vi "Phase Tune.vi"(11 "Hardware Parameters":T1={"Scan Calibration [G/V]"=0.0, "Modulation Calibration [G/V]"=0.0, "Modulation Phase [deg]"=0.0, "Modulation Frequency [Hz]"=0.0, "Attenuation [dB]"=0, "Input Channel Count"=0, "Time constant"=7, "Sensitivity"=17, "Frequency Output Voltage [V]"=0.0, "Phase Output Voltage [V]"=0.0, "Lock-in Offset Compensation"=FALSE, "RF [GHz]"=0.0, "Q Start"=0.0, "Q End"=0.0, "Balance"=0.0, "Phase Error"=0.0, "AFC Error"=0.0, "AFC"=FALSE, "Magnet Rotation"=FALSE, "Balance Scaling Factor"=1.0, "Phase Error Scaling Factor"=1.0, "AFC Error Scaling Factor"=1.0, "Frequency Counter ID"="", "Sweep Waveform"=enum."Sawtooth", "Q-Factor Scale"=0.0, " Q-Data Scale"=0.0, " Q-Data Offset"=0.0, "Magnet Rotation Slope"=0.0, "Magnet Rotation Offset"=0.0, "Phase Sweep Resolution"=0.0, "Hardware Version Number"="", "Spectrometer ID Number"=0, "Spectrometer Name"="", "Lock in Saturation"=0.0, "Balance Threshold"=0.0, "Phase Error Threshold"=0.0, "AFC Error Threshold"=0.0, "Linear Actuator Length"=0.0, "Lock-in OK?"=FALSE, "Ignore Lock-in Comm. Failure"=FALSE, "Gradient Addresses"=[], "Gradient Calibrations [G/A*mm]"=[], "Gradient Power Supplies"=[], "Lock-in Address"="", "Magnet Type"=enum."RRI", "Camera Names"=[], "Sweep Limit [Gauss]"=0.0, "Modulation Limit [Gauss]"=0.0, "Balance Threshold Exceeded?"=FALSE, "Phase Threshold Exceeded?"=FALSE, "AFC Threshold Exceeded?"=FALSE, "Consecutive Re-tune attempts"=0, "Reverse Sweep Slope [sec]"=0.0, "Reverse Sweep Offset [G]"=0.0, "AFC Field Correction [V/MHz]"=0.0, "Active Gradients (X Y Z)"=[], "SpO2 Calibration [SpO2/V]"=1.0, "Heart Rate Calibration [BPM/V]"=1.0, "Thermocouple Channel"=""} {"Sensitivity" items=["", "2 nV", "5 nV", "10 nV", "20 nV", "50 nV", "100 nV", "200 nV", "500 nV", "1 uV", "2 uV", "5 uV", "10 uV", "20 uV", "50 uV", "100 uV", "200 uV", "500 uV", "1 mV", "2 mV", "5 mV", "10 mV", "20 mV", "50 mV", "100 mV", "200 mV", "500 mV", "1 V"]; "Time constant" items=["10 us", "20 us", "40 us", "80 us", "160 us", "320 us", "640 us", "5 ms", "10 ms", "20 ms", "50 ms", "100 ms", "200 ms", "500 ms", "1 s", "2 s", "5 s", "10 s", "20 s", "50 s", "100 s", "200 s", "500 s", "1 ks", "2 ks", "5 ks", "10 ks", "20 ks", "50 ks", "100 ks"]}) -> (1 "Phase Threshold Exceeded":bool, 2 "Phase Voltage [v]":dbl, 3 "Hardware Parameters Out":T1={"Scan Calibration [G/V]"=0.0, "Modulation Calibration [G/V]"=0.0, "Modulation Phase [deg]"=0.0, "Modulation Frequency [Hz]"=0.0, "Attenuation [dB]"=0, "Input Channel Count"=0, "Time constant"=7, "Sensitivity"=17, "Frequency Output Voltage [V]"=0.0, "Phase Output Voltage [V]"=0.0, "Lock-in Offset Compensation"=FALSE, "RF [GHz]"=0.0, "Q Start"=0.0, "Q End"=0.0, "Balance"=0.0, "Phase Error"=0.0, "AFC Error"=0.0, "AFC"=FALSE, "Magnet Rotation"=FALSE, "Balance Scaling Factor"=1.0, "Phase Error Scaling Factor"=1.0, "AFC Error Scaling Factor"=1.0, "Frequency Counter ID"="", "Sweep Waveform"=enum."Sawtooth", "Q-Factor Scale"=0.0, " Q-Data Scale"=0.0, " Q-Data Offset"=0.0, "Magnet Rotation Slope"=0.0, "Magnet Rotation Offset"=0.0, "Phase Sweep Resolution"=0.0, "Hardware Version Number"="", "Spectrometer ID Number"=0, "Spectrometer Name"="", "Lock in Saturation"=0.0, "Balance Threshold"=0.0, "Phase Error Threshold"=0.0, "AFC Error Threshold"=0.0, "Linear Actuator Length"=0.0, "Lock-in OK?"=FALSE, "Ignore Lock-in Comm. Failure"=FALSE, "Gradient Addresses"=[], "Gradient Calibrations [G/A*mm]"=[], "Gradient Power Supplies"=[], "Lock-in Address"="", "Magnet Type"=enum."RRI", "Camera Names"=[], "Sweep Limit [Gauss]"=0.0, "Modulation Limit [Gauss]"=0.0, "Balance Threshold Exceeded?"=FALSE, "Phase Threshold Exceeded?"=FALSE, "AFC Threshold Exceeded?"=FALSE, "Consecutive Re-tune attempts"=0, "Reverse Sweep Slope [sec]"=0.0, "Reverse Sweep Offset [G]"=0.0, "AFC Field Correction [V/MHz]"=0.0, "Active Gradients (X Y Z)"=[], "SpO2 Calibration [SpO2/V]"=1.0, "Heart Rate Calibration [BPM/V]"=1.0, "Thermocouple Channel"=""} {"Sensitivity" items=["", "2 nV", "5 nV", "10 nV", "20 nV", "50 nV", "100 nV", "200 nV", "500 nV", "1 uV", "2 uV", "5 uV", "10 uV", "20 uV", "50 uV", "100 uV", "200 uV", "500 uV", "1 mV", "2 mV", "5 mV", "10 mV", "20 mV", "50 mV", "100 mV", "200 mV", "500 mV", "1 V"]; "Time constant" items=["10 us", "20 us", "40 us", "80 us", "160 us", "320 us", "640 us", "5 ms", "10 ms", "20 ms", "50 ms", "100 ms", "200 ms", "500 ms", "1 s", "2 s", "5 s", "10 s", "20 s", "50 s", "100 s", "200 s", "500 s", "1 ks", "2 ks", "5 ks", "10 ks", "20 ks", "50 ks", "100 ks"]})   [LabVIEW 2016]
uses:
  Types/Hardware Parameters.ctl
panel:
  out "min index stg2":i32=90
  out "min value stg2":dbl=0.00457763671875
  out "min value":dbl=0.0262451171875
  out "min index(es)":i32=11
  in  "SpanSTG1":dbl=20000.0
  in  "EndThresh":dbl
  out "localMinima":dbl
  in  "stg2Begin":i32
  out "stg2End":i32=90
  in  "#StepsSTG2":u32=128
  in  "setBack1":i32=4
  out "STG2Offset":dbl=-7187.5
  in  "SpanSTG2":dbl=1000.0
  out "STG2ExcitationArray":dbl[](array[numeric])=[-7687.5, -7679.6875, -7671.875, -7664.0625, -7656.25, -7648.4375, -7640.625, -7632.8125, -7625.0, -7617.1875, -7609.375, -7601.5625, -7593.75, -7585.9375, -7578.125, -7570.3125, -7562.5, -7554.6875, -7546.875, -7539.0625, -7531.25, -7523.4375, -7515.625, -7507.8125, -7500.0, -7492.1875, -7484.375, -7476.5625, -7468.75, -7460.9375, -7453.125, -7445.3125, -7437.5, -7429.6875, -7421.875, -7414.0625, -7406.25, -7398.4375, -7390.625, -7382.8125, -7375.0, -7367.1875, -7359.375, -7351.5625, -7343.75, -7335.9375, -7328.125, -7320.3125, -7312.5, -7304.6875, -7296.875, -7289.0625, -7281.25, -7273.4375, -7265.625, -7257.8125, -7250.0, -7242.1875, -7234.375, -7226.5625, -7218.75, -7210.9375, -7203.125, -7195.3125, -7187.5, -7179.6875, -7171.875, -7164.0625, -7156.25, -7148.4375, -7140.625, -7132.8125, -7125.0, -7117.1875, -7109.375, -7101.5625, -7093.75, -7085.9375, -7078.125, -7070.3125, -7062.5, -7054.6875, -7046.875, -7039.0625, -7031.25, -7023.4375, -7015.625, -7007.8125, -7000.0, -6992.1875, -6984.375, -6976.5625, -6968.75, -6960.9375, -6953.125, -6945.3125, -6937.5, -6929.6875, -6921.875, -6914.0625, -6906.25, -6898.4375, -6890.625, -6882.8125, -6875.0, -6867.1875, -6859.375, -6851.5625, -6843.75, -6835.9375, -6828.125, -6820.3125, -6812.5, -6804.6875, -6796.875, -6789.0625, -6781.25, -6773.4375, -6765.625, -6757.8125, -6750.0, -6742.1875, -6734.375, -6726.5625, -6718.75, -6710.9375, -6703.125, -6695.3125]
  in  "stg1End":i32=11
  out "StableIncreaseFound":bool
  out "StableDecreaseFound":bool
  out "ExcitationArray":dbl[](array[numeric])=[-10000.0, -9687.5, -9375.0, -9062.5, -8750.0, -8437.5, -8125.0, -7812.5, -7500.0, -7187.5, -6875.0, -6562.5, -6250.0, -5937.5, -5625.0, -5312.5, -5000.0, -4687.5, -4375.0, -4062.5, -3750.0, -3437.5, -3125.0, -2812.5, -2500.0, -2187.5, -1875.0, -1562.5, -1250.0, -937.5, -625.0, -312.5, 0.0, 312.5, 625.0, 937.5, 1250.0, 1562.5, 1875.0, 2187.5, 2500.0, 2812.5, 3125.0, 3437.5, 3750.0, 4062.5, 4375.0, 4687.5, 5000.0, 5312.5, 5625.0, 5937.5, 6250.0, 6562.5, 6875.0, 7187.5, 7500.0, 7812.5, 8125.0, 8437.5, 8750.0, 9062.5, 9375.0, 9687.5, 10000.0] format="%#_12g"
  in  "#StepsSTG1":u32=64
  out "XY Graph":cluster{"Y":dbl[], "Y":dbl[]}[](graph)=[{"Y"=[0.0, 1.0, 2.0, 3.0, 4.0, 5.0, 6.0, 7.0, 8.0, 9.0, 10.0, 11.0, 12.0, 13.0, 14.0, 15.0, 16.0, 17.0, 18.0, 19.0, 20.0, 21.0, 22.0, 23.0, 24.0, 25.0, 26.0, 27.0, 28.0, 29.0, 30.0, 31.0, 32.0, 33.0, 34.0, 35.0, 36.0, 37.0, 38.0, 39.0, 40.0, 41.0, 42.0, 43.0, 44.0, 45.0, 46.0, 47.0, 48.0, 49.0, 50.0, 51.0, 52.0, 53.0, 54.0, 55.0, 56.0, 57.0, 58.0, 59.0, 60.0, 61.0, 62.0, 63.0, 64.0, 65.0, 66.0, 67.0, 68.0, 69.0, 70.0, 71.0, 72.0, 73.0, 74.0, 75.0, 76.0, 77.0, 78.0, 79.0, 80.0, 81.0, 82.0, 83.0, 84.0, 85.0, 86.0, 87.0, 88.0, 89.0, 90.0, 91.0, 92.0, 93.0, 94.0, 95.0, 96.0, 97.0, 98.0, 99.0, 100.0, 101.0, 102.0, 103.0, 104.0, 105.0, 106.0, 107.0, 108.0, 109.0, 110.0, 111.0, 112.0, 113.0, 114.0, 115.0, 116.0, 117.0, 118.0, 119.0, 120.0, 121.0, 122.0, 123.0, 124.0, 125.0, 126.0, 127.0, 128.0], "Y"=[1.0369873046875, 1.0302734375, 1.00128173828125, 0.99609375, 0.96099853515625, 0.95733642578125, 0.938720703125, 0.91522216796875, 0.9051513671875, 0.8734130859375, 0.8685302734375, 0.83892822265625, 0.8319091796875, 0.8209228515625, 0.81695556640625, 0.7861328125, 0.76690673828125, 0.74462890625, 0.71868896484375, 0.71380615234375, 0.6744384765625, 0.67291259765625, 0.65277099609375, 0.65155029296875, 0.62103271484375, 0.5950927734375, 0.58441162109375, 0.5517578125, 0.548095703125, 0.531005859375, 0.528564453125, 0.49774169921875, 0.482177734375, 0.457763671875, 0.43182373046875, 0.42205810546875, 0.39031982421875, 0.386962890625, 0.369873046875, 0.3558349609375, 0.33233642578125, 0.30548095703125, 0.2996826171875, 0.26611328125, 0.262451171875, 0.22552490234375, 0.22369384765625, 0.21148681640625, 0.18310546875, 0.167236328125, 0.14190673828125, 0.1336669921875, 0.1043701171875, 0.09918212890625, 0.06591796875, 0.04547119140625, 0.0384521484375, 0.0262451171875, 0.00457763671875, 0.01068115234375, 0.04302978515625, 0.0439453125, 0.06561279296875, 0.09124755859375, 0.10406494140625, 0.1336669921875, 0.13641357421875, 0.16876220703125, 0.17059326171875, 0.18707275390625, 0.19622802734375, 0.22796630859375, 0.24322509765625, 0.2606201171875, 0.29815673828125, 0.30029296875, 0.32012939453125, 0.3271484375, 0.3533935546875, 0.36285400390625, 0.390625, 0.41748046875, 0.42999267578125, 0.44219970703125, 0.44403076171875, 0.478515625, 0.49591064453125, 0.5194091796875, 0.54656982421875, 0.5560302734375, 0.5859375, 0.594482421875, 0.6298828125, 0.63323974609375, 0.64727783203125, 0.67291259765625, 0.68511962890625]}]
  # "Bridge I/O"
  # "Magnet Rotation"
  # "Field Calibration"
  # "Lock In Amplifier"
  # "Spectrometer Information"
  # "DAQ Settings"
  # "Gradient Coils and Field"
  # "X"
  # "Y"
  # "Z"
  # "Q-Measurements"
  # "Bridge I/O"
  # "Magnet Rotation"
  # "Field Calibration"
  # "Lock In Amplifier"
  # "Spectrometer Information"
  # "DAQ Settings"
  # "Gradient Coils and Field"
  # "X"
  # "Y"
  # "Z"
  # "Q-Measurements"
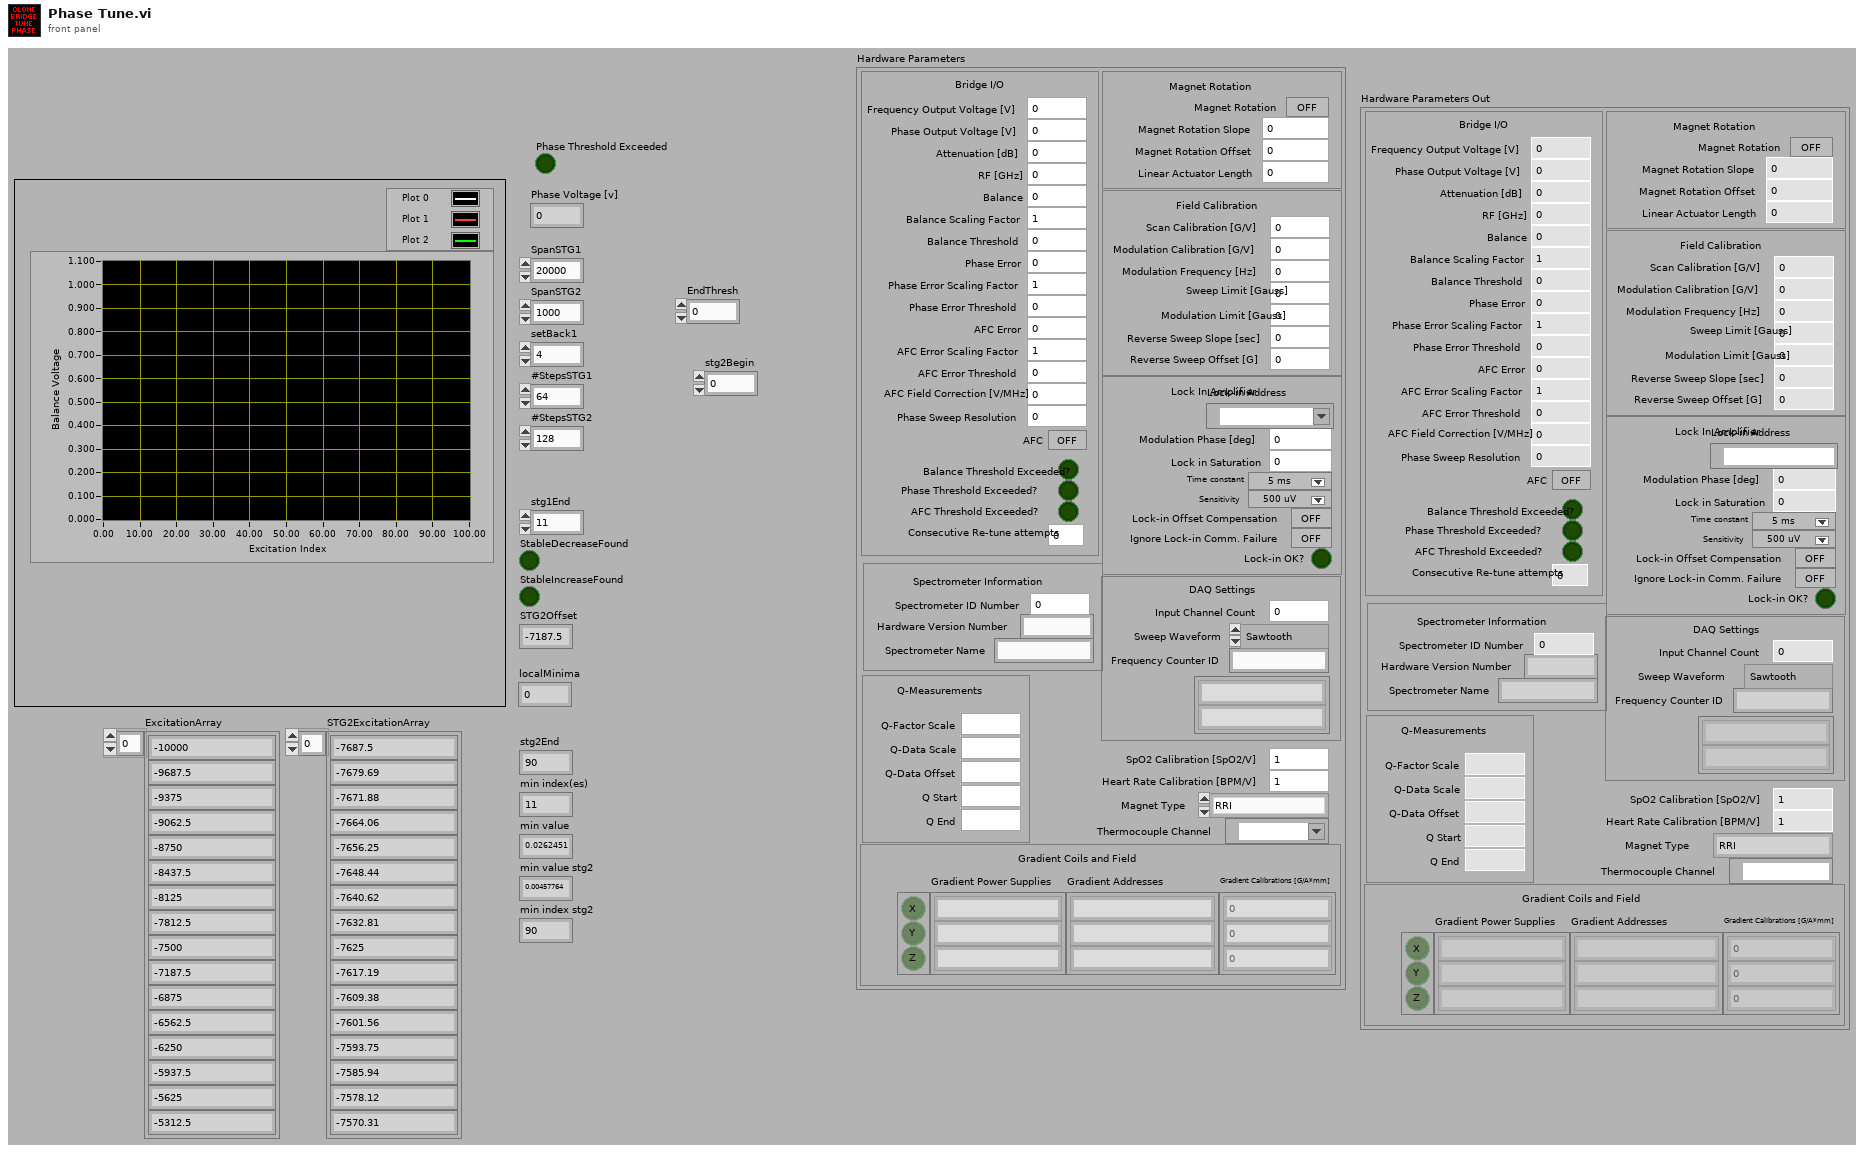
[diagram p1: front panel]
types:
  T1 = typedef "Hardware Parameters.ctl" = cluster{"Scan Calibration [G/V]":dbl, "Modulation Calibration [G/V]":dbl, "Modulation Phase [deg]":dbl, "Modulation Frequency [Hz]":dbl, "Attenuation [dB]":u16, "Input Channel Count":i32, "Time constant":u16, "Sensitivity":u16, "Frequency Output Voltage [V]":dbl, "Phase Output Voltage [V]":dbl, "Lock-in Offset Compensation":bool, "RF [GHz]":dbl, "Q Start":dbl, "Q End":dbl, "Balance":dbl, "Phase Error":dbl, "AFC Error":dbl, "AFC":bool, "Magnet Rotation":bool, "Balance Scaling Factor":dbl, "Phase Error Scaling Factor":dbl, "AFC Error Scaling Factor":dbl, "Frequency Counter ID":string, "Sweep Waveform":enum16{"Sine Wave", "Square Wave", "Sawtooth", "Triangle Wave"}, "Q-Factor Scale":dbl, " Q-Data Scale":dbl, " Q-Data Offset":dbl, "Magnet Rotation Slope":dbl, "Magnet Rotation Offset":dbl, "Phase Sweep Resolution":dbl, "Hardware Version Number":string, "Spectrometer ID Number":i32, "Spectrometer Name":string, "Lock in Saturation":dbl, "Balance Threshold":dbl, "Phase Error Threshold":dbl, "AFC Error Threshold":dbl, "Linear Actuator Length":dbl, "Lock-in OK?":bool, "Ignore Lock-in Comm. Failure":bool, "Gradient Addresses":string[], "Gradient Calibrations [G/A*mm]":dbl[], "Gradient Power Supplies":string[], "Lock-in Address":refnum<visa-resource-name>, "Magnet Type":enum16{"RRI", "BARDA", "Whole Body Permanent", "RRI Electromagnet"}, "Camera Names":string[], "Sweep Limit [Gauss]":dbl, "Modulation Limit [Gauss]":dbl, "Balance Threshold Exceeded?":bool, "Phase Threshold Exceeded?":bool, "AFC Threshold Exceeded?":bool, "Consecutive Re-tune attempts":i32, "Reverse Sweep Slope [sec]":dbl, "Reverse Sweep Offset [G]":dbl, "AFC Field Correction [V/MHz]":dbl, "Active Gradients (X Y Z)":bool[], "SpO2 Calibration [SpO2/V]":dbl, "Heart Rate Calibration [BPM/V]":dbl, "Thermocouple Channel":tag}
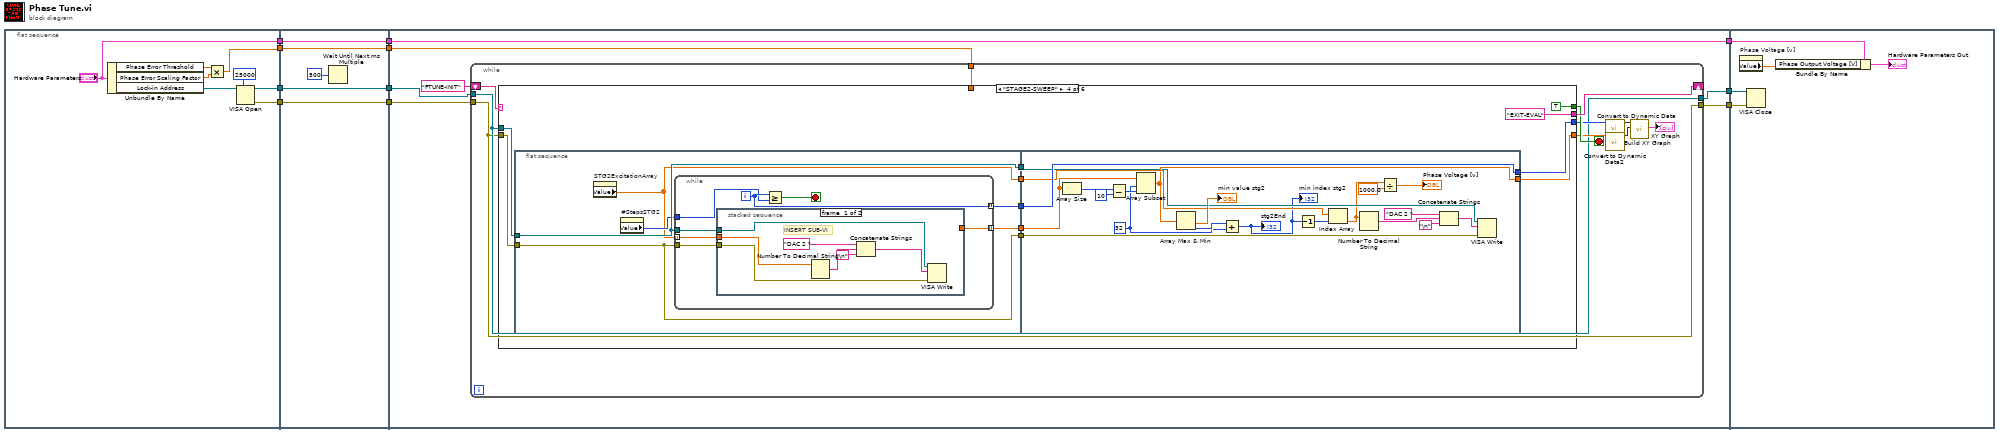
[diagram p0: block diagram]
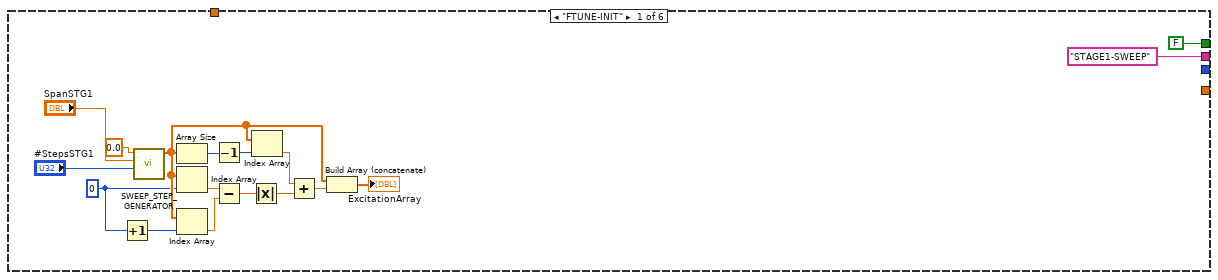
[diagram p2: hidden frame]
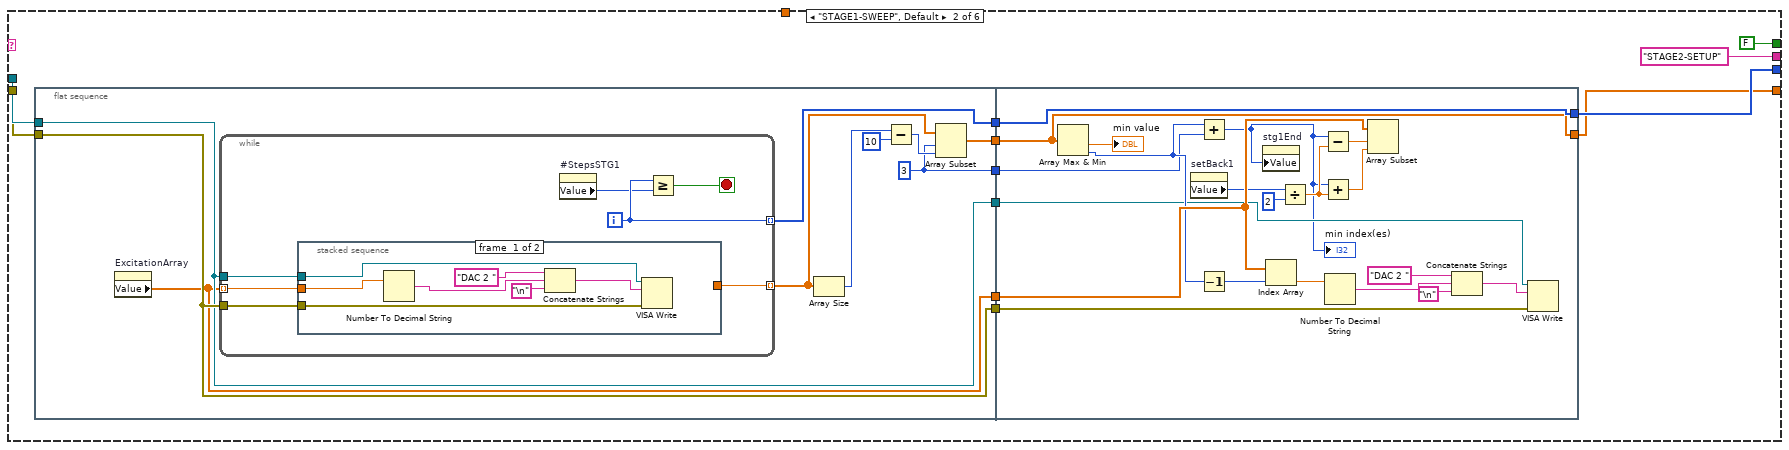
[diagram p3: hidden frame]
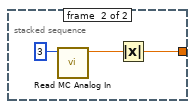
[diagram p4: hidden frame]
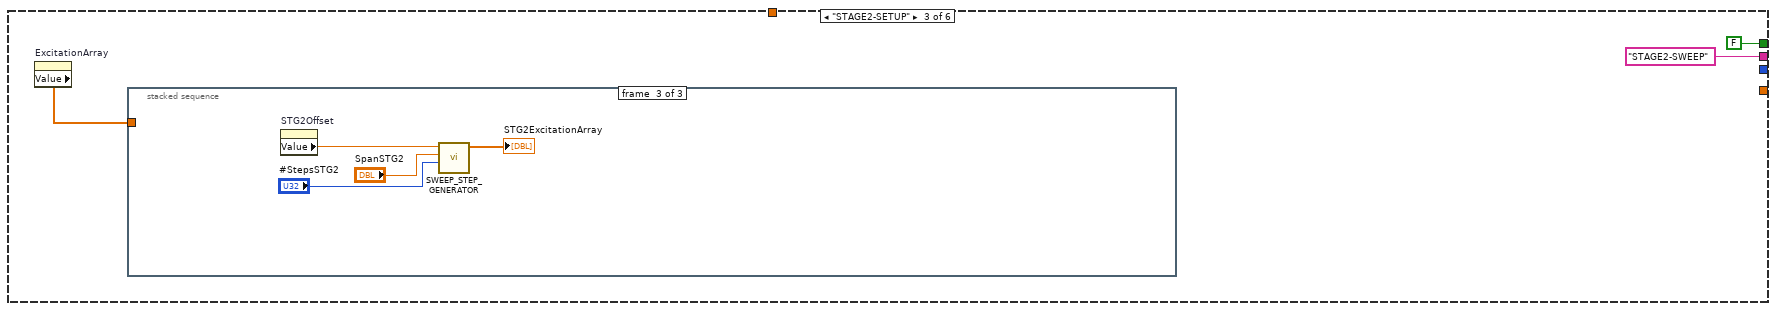
[diagram p5: hidden frame]
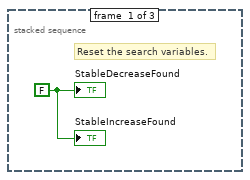
[diagram p6: hidden frame]
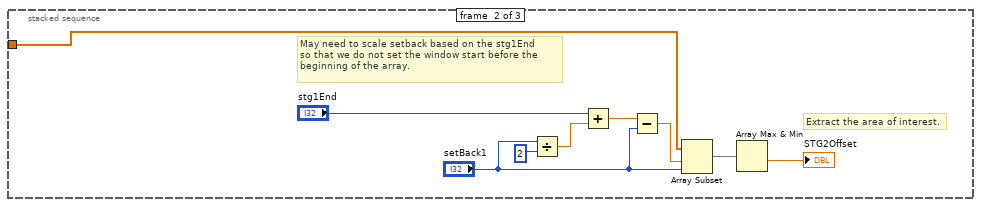
[diagram p7: hidden frame]
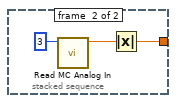
[diagram p8: hidden frame]
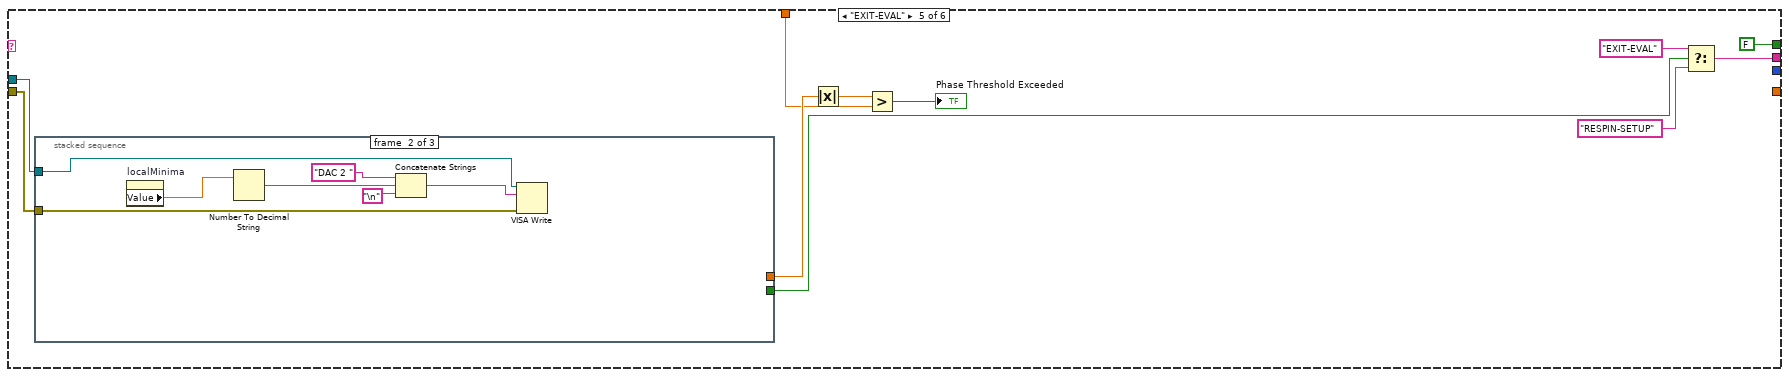
[diagram p9: hidden frame]
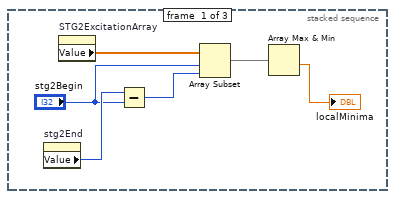
[diagram p10: hidden frame]
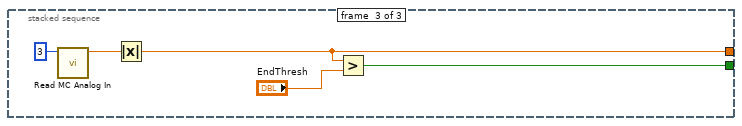
[diagram p11: hidden frame]
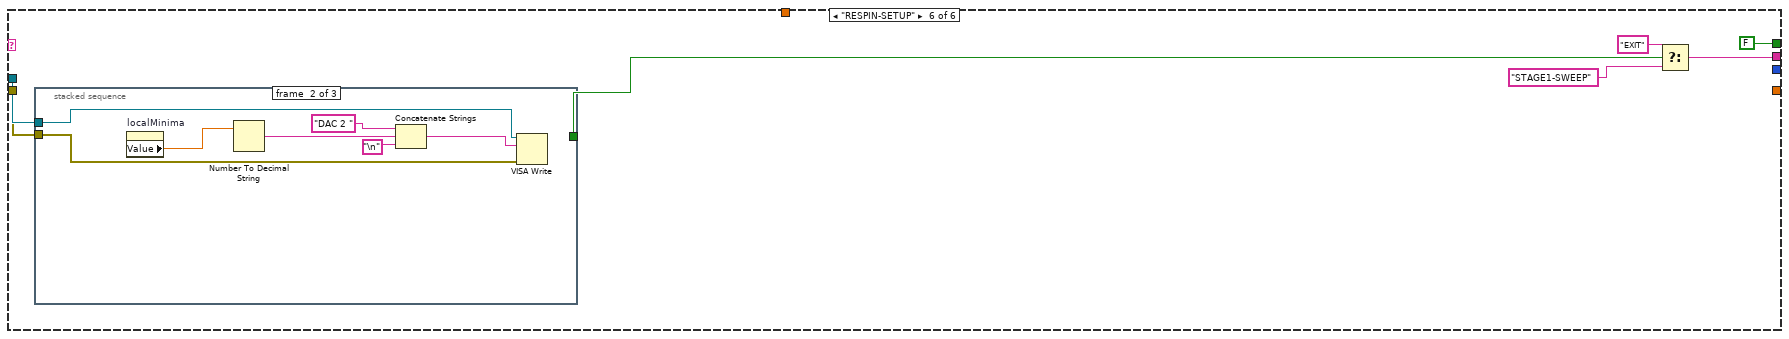
[diagram p12: hidden frame]
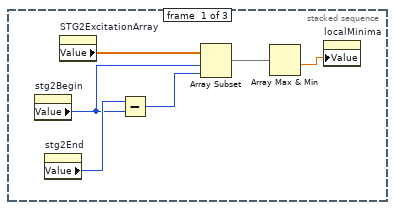
[diagram p13: hidden frame]
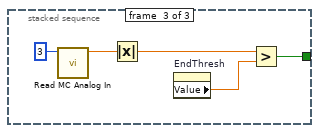
[diagram p14: hidden frame]
diagram:
  n1 = flat-sequence {
    tunnel: [w14] -> w6
    tunnel: [w15] -> w5
    tunnel: [w13] -> w4
    tunnel: ["Hardware Parameters"] -> w1
    tunnel: [w24] -> w9
    tunnel: [w23] -> w8
    tunnel: [w22] -> w7
    tunnel: w6 -> [w24]
    tunnel: w5 -> [w22]
    tunnel: w4 -> [w23]
    tunnel: [w20] -> w2
    tunnel: w1 -> [w20]
    tunnel: [w28] -> w11
    tunnel: [w27] -> w10
    tunnel: w9 -> [w30]
    tunnel: w8 -> [w29]
    tunnel: w7 -> [w26]
    tunnel: [w25] -> w3
    tunnel: w2 -> [w25]
    tunnel: w11 -> [w249]
    tunnel: w10 -> [w248]
    tunnel: w3 -> [w246]
    frame #0 {
      n2 = Unbundle By Name("Hardware Parameters") -> ("Phase Error Threshold"=w19:dbl, "Phase Error Scaling Factor"=w18:dbl, "Lock-in Address"=w17:refnum<visa-resource-name>)
      n3 = Multiply(x=w19, y=w18) -> (x*y=w15:dbl)
      n4 = VISA Open(timeout (0)=u32 25000 ("VISA Open timeout (0)"), VISA resource name=w17) -> (VISA resource name=w14:refnum<visa-resource-name>, error out=w13:errorcluster)  [unwired: 1 in, 2 out]
    }
    frame #1 {
      n5 = Wait Until Next ms Multiple(millisecond multiple=u32 500) -> ()  [unwired: 1 out]
    }
    frame #2 {
      n6 = while {
        shift-right: [w41] -> _
        shift-left: "FTUNE-INIT" -> [w42]
        tunnel: w30 -> [w34]
        tunnel: w29 -> [w33]
        tunnel: [w34] -> w28
        tunnel: [w33] -> w27
        tunnel: w26 -> [w32]
        stop <- w40 stop-if-true
        n7 = case shown="\"STAGE2-SWEEP\"" w42 {
          tunnel: ["STAGE1-SWEEP" "STAGE2-SETUP" "STAGE2-SWEEP" "EXIT-EVAL" w199 w224] -> w41
          tunnel: [FALSE FALSE FALSE TRUE FALSE FALSE] -> w40
          tunnel: [_ w69 _ w140 _ _] -> w36
          tunnel: [_ w68 _ w141 _ _] -> w35
          tunnel: w34 -> [_ w64 _ w139 w196 w221]
          tunnel: w33 -> [_ w63 _ w137 w195 w220]
          tunnel: w32 -> [_ _ _ _ w191 _]
          frame "FTUNE-INIT" {
            w47 = 0 ("index")
            n8 = Increment(x=w47) -> (x+1=w48:i32)
            n9 = call "SWEEP_STEP_GENERATOR.vi"("STEPS"="#StepsSTG1", "SPAN"="SpanSTG1", "OFFSET"=0.0) -> ("SteppedArrayOut"=w49:dbl[])  [unwired: 6 in, 2 out]
            n10 = Array Size(array=w49) -> (size(s)=w53:i32)
            n11 = Index Array(array=w49, index=w47) -> (element=w56:dbl)
            n12 = Index Array(array=w49, index=w48) -> (element=w55:dbl)
            n13 = Decrement(x=w53) -> (x-1=w46:i32)
            n14 = Subtract(x=w56, y=w55) -> (x-y=w54:dbl)
            n15 = Absolute Value(x=w54) -> (abs(x)=w51:dbl)
            n16 = Index Array(array=w49, index=w46) -> (element=w52:dbl)
            n17 = Add(x=w52, y=w51) -> (x+y=w50:dbl)
            n18 = Build Array (concatenate)(w49, w50) -> (→"ExcitationArray":dbl[])
          }
          frame "STAGE1-SWEEP", Default {
            n19 = flat-sequence {
              tunnel: [w81] -> w67
              tunnel: [w78] -> w66
              tunnel: [w72] -> w65
              tunnel: w64 -> [w79]
              tunnel: w63 -> [w80]
              tunnel: [w80] -> w62
              tunnel: [w79] -> w61
              tunnel: [w73] -> w60
              tunnel: [w112] -> w68
              tunnel: [w118] -> w69
              tunnel: w67 -> [w118]
              tunnel: w66 -> [w112]
              tunnel: w65 -> [w111]
              tunnel: w62 -> [w107]
              tunnel: w61 -> [w106]
              tunnel: w60 -> [w105]
              frame #0 {
                w73 = 3 ("index")
                n20 = property on="ExcitationArray" class="Arr (strict)"() -> ("Value"=w72:dbl[])  [unwired: 2 in, 2 out]
                n21 = while {
                  tunnel: w72 -> [w86] mode=indexing
                  tunnel: [w88] -> w81 mode=indexing
                  tunnel: [w85] -> w77 mode=indexing
                  tunnel: w79 -> [w84]
                  tunnel: w80 -> [w83]
                  i -> [w88]
                  stop <- w87 stop-if-true
                  n22 = stacked-sequence {
                    tunnel: w86 -> [w91 _]
                    tunnel: [_ w98] -> w85
                    tunnel: w84 -> [w89 _]
                    tunnel: w83 -> [w90 _]
                    frame #0 {
                      n23 = Number To Decimal String(number=w91) -> (decimal integer string=w95:string)  [unwired: 1 out]
                      n24 = Concatenate Strings("DAC 2 " ("write buffer"), w95, "\n") -> (w92:string)
                      n25 = VISA Write(VISA resource name=w89, write buffer=w92, error in (no error)=w90) -> ()  [unwired: 3 out]
                    }
                    frame #1 {
                      n26 = call "Read MC Analog In.vi"("channel"=3) -> ("Voltage Input"=w96:dbl)  [unwired: 9 in, 1 out]
                      n27 = Absolute Value(x=w96) -> (abs(x)=w98:dbl)
                    }
                  }
                  n28 = property on="#StepsSTG1" class="DigNum (strict)"() -> ("Value"=w82:u32)  [unwired: 2 in, 2 out]
                  n29 = Greater Or Equal?(x=w88, y=w82) -> (x >= y?=w87:bool)
                }
                n30 = Array Size(array=w77) -> (size(s)=w76:i32)
                n31 = Subtract(x=w76, y=10) -> (x-y=w74:i32)
                n32 = Array Subset(array=w77, index=w73, length=w74) -> (w78:dbl[])
              }
              frame #1 {
                n33 = Array Max & Min(array=w112) -> (min value=→"min value":dbl, min index (indices)=w108:i32)  [unwired: 2 out]
                n34 = property on="setBack1" class="DigNum (strict)"() -> ("Value"=w99:i32)  [unwired: 2 in, 2 out]
                n35 = Add(x=w108, y=w105) -> (x+y=w100:i32)
                "min index(es)" <- w100
                n36 = Decrement(x=w108) -> (x-1=w109:i32)
                n37 = property on="stg1End" class="DigNum (strict)"("Value"=w100) -> ()  [unwired: 2 in, 2 out]
                n38 = Index Array(array=w111, index=w109) -> (element=w110:dbl)
                n39 = Divide(x=w99, y=2) -> (x/y=w114:dbl)
                n40 = Subtract(x=w100, y=w114) -> (x-y=w117:dbl)
                n41 = Add(x=w100, y=w114) -> (x+y=w116:dbl)
                n42 = Number To Decimal String(number=w110) -> (decimal integer string=w104:string)  [unwired: 1 out]
                n43 = Array Subset(array=w111, index=w117, length=w116) -> ()  [unwired: 1 out]
                n44 = Concatenate Strings("DAC 2 " ("write buffer"), w104, "\n") -> (w101:string)
                n45 = VISA Write(VISA resource name=w106, write buffer=w101, error in (no error)=w107) -> ()  [unwired: 3 out]
              }
            }
          }
          frame "STAGE2-SETUP" {
            n46 = property on="ExcitationArray" class="Arr (strict)"() -> ("Value"=w119:dbl[])  [unwired: 2 in, 2 out]
            n47 = stacked-sequence {
              tunnel: w119 -> [_ w131 _]
              frame #0 {
                w122 = FALSE ("StableIncreaseFound")
                # "Reset the search variables."
                "StableDecreaseFound" <- w122
                "StableIncreaseFound" <- w122
              }
              frame #1 {
                # "May need to scale setback based on the stg1End\nso that we do not set the window start before the \nbeginning of the array."
                # "Extract the area of interest."
                n48 = Divide(x="setBack1", y=2) -> (x/y=w126:dbl)
                n49 = Add(x="stg1End", y=w126) -> (x+y=w128:dbl)
                n50 = Subtract(x=w128, y="setBack1") -> (x-y=w130:dbl)
                n51 = Array Subset(array=w131, index=w130, length="setBack1") -> (w129:dbl[])
                n52 = Array Max & Min(array=w129) -> (min value=→"STG2Offset":dbl)  [unwired: 3 out]
              }
              frame #2 {
                n53 = property on="STG2Offset" class="DigNum (strict)"() -> ("Value"=w132:dbl)  [unwired: 2 in, 2 out]
                n54 = call "SWEEP_STEP_GENERATOR.vi"("STEPS"="#StepsSTG2", "SPAN"="SpanSTG2", "OFFSET"=w132) -> ("SteppedArrayOut"=→"STG2ExcitationArray":dbl[])  [unwired: 6 in, 2 out]
              }
            }
          }
          frame "STAGE2-SWEEP" {
            n55 = flat-sequence {
              tunnel: [w152] -> w144
              tunnel: [w151] -> w143
              tunnel: [w147] -> w142
              tunnel: w139 -> [w150]
              tunnel: [w150] -> w138
              tunnel: w137 -> [w149]
              tunnel: [w149] -> w136
              tunnel: [w181] -> w141
              tunnel: [w190] -> w140
              tunnel: w144 -> [w190]
              tunnel: w143 -> [w182]
              tunnel: w142 -> [w183]
              tunnel: w138 -> [w179]
              tunnel: w136 -> [w178]
              frame #0 {
                n56 = property on="STG2ExcitationArray" class="Arr (strict)"() -> ("Value"=w147:dbl[])  [unwired: 2 in, 2 out]
                n57 = property on="#StepsSTG2" class="DigNum (strict)"() -> ("Value"=w148:u32)  [unwired: 2 in, 2 out]
                n58 = while {
                  tunnel: w147 -> [w157] mode=indexing
                  tunnel: [w159] -> w152 mode=indexing
                  tunnel: [w156] -> w151 mode=indexing
                  tunnel: w150 -> [w155]
                  tunnel: w149 -> [w154]
                  tunnel: w148 -> [w153]
                  i -> [w159]
                  stop <- w158 stop-if-true
                  n59 = stacked-sequence {
                    tunnel: w157 -> [w166 _]
                    tunnel: [_ w169] -> w156
                    tunnel: w155 -> [w165 _]
                    tunnel: w154 -> [w164 _]
                    frame #0 {
                      # "INSERT SUB-VI"
                      n60 = Number To Decimal String(number=w166) -> (decimal integer string=w161:string)  [unwired: 1 out]
                      n61 = Concatenate Strings("DAC 2 " ("write buffer"), w161, "\n") -> (w160:string)
                      n62 = VISA Write(VISA resource name=w165, write buffer=w160, error in (no error)=w164) -> ()  [unwired: 3 out]
                    }
                    frame #1 {
                      n63 = call "Read MC Analog In.vi"("channel"=3) -> ("Voltage Input"=w167:dbl)  [unwired: 9 in, 1 out]
                      n64 = Absolute Value(x=w167) -> (abs(x)=w169:dbl)
                    }
                  }
                  n65 = Greater Or Equal?(x=w159, y=w153) -> (x >= y?=w158:bool)
                }
              }
              frame #1 {
                w180 = 32 ("index")
                n66 = Array Size(array=w182) -> (size(s)=w186:i32)
                n67 = Subtract(x=w186, y=10) -> (x-y=w184:i32)
                n68 = Array Subset(array=w182, index=w180, length=w184) -> (w181:dbl[])
                n69 = Array Max & Min(array=w181) -> (min value=→"min value stg2":dbl, min index (indices)=w187:i32)  [unwired: 2 out]
                n70 = Add(x=w187, y=w180) -> (x+y=w170:i32)
                "min index stg2" <- w170
                "stg2End" <- w170
                n71 = Decrement(x=w170) -> (x-1=w188:i32)
                n72 = Index Array(array=w183, index=w188) -> (element=w177:dbl)
                n73 = Number To Decimal String(number=w177) -> (decimal integer string=w172:string)  [unwired: 1 out]
                n74 = Divide(x=w177, y=1000.0) -> (x/y=→"Phase Voltage [v]":dbl)
                n75 = Concatenate Strings("DAC 2 " ("write buffer"), w172, "\n") -> (w171:string)
                n76 = VISA Write(VISA resource name=w179, write buffer=w171, error in (no error)=w178) -> ()  [unwired: 3 out]
              }
            }
          }
          frame "EXIT-EVAL" {
            n77 = stacked-sequence {
              tunnel: [_ _ w219] -> w197
              tunnel: w196 -> [_ w214 _]
              tunnel: w195 -> [_ w213 _]
              tunnel: [_ _ w215] -> w193
              frame #0 {
                n78 = property on="stg2End" class="DigNum (strict)"() -> ("Value"=w204:i32)  [unwired: 2 in, 2 out]
                n79 = property on="STG2ExcitationArray" class="Arr (strict)"() -> ("Value"=w205:dbl[])  [unwired: 2 in, 2 out]
                n80 = Subtract(x=w204, y="stg2Begin") -> (x-y=w207:i32)
                n81 = Array Subset(array=w205, index="stg2Begin", length=w207) -> (w206:dbl[])
                n82 = Array Max & Min(array=w206) -> (min value=→"localMinima":dbl)  [unwired: 3 out]
              }
              frame #1 {
                n83 = property on="localMinima" class="DigNum (strict)"() -> ("Value"=w208:dbl)  [unwired: 2 in, 2 out]
                n84 = Number To Decimal String(number=w208) -> (decimal integer string=w210:string)  [unwired: 1 out]
                n85 = Concatenate Strings("DAC 2 " ("write buffer"), w210, "\n") -> (w209:string)
                n86 = VISA Write(VISA resource name=w214, write buffer=w209, error in (no error)=w213) -> ()  [unwired: 3 out]
              }
              frame #2 {
                n87 = call "Read MC Analog In.vi"("channel"=3) -> ("Voltage Input"=w216:dbl)  [unwired: 9 in, 1 out]
                n88 = Absolute Value(x=w216) -> (abs(x)=w215:dbl)
                n89 = Greater?(x=w215, y="EndThresh") -> (0:w219:bool)
              }
            }
            n90 = Absolute Value(x=w193) -> (abs(x)=w192:dbl)
            n91 = Greater?(x=w192, y=w191) -> (0:→"Phase Threshold Exceeded":bool)
            n92 = Select(t="EXIT-EVAL", s=w197, f="RESPIN-SETUP") -> (s? t:f=w199:string)
          }
          frame "RESPIN-SETUP" {
            n93 = stacked-sequence {
              tunnel: [_ _ w243] -> w222
              tunnel: w221 -> [_ w239 _]
              tunnel: w220 -> [_ w238 _]
              frame #0 {
                n94 = property on="stg2Begin" class="DigNum (strict)"() -> ("Value"=w228:i32)  [unwired: 2 in, 2 out]
                n95 = property on="stg2End" class="DigNum (strict)"() -> ("Value"=w229:i32)  [unwired: 2 in, 2 out]
                n96 = property on="STG2ExcitationArray" class="Arr (strict)"() -> ("Value"=w230:dbl[])  [unwired: 2 in, 2 out]
                n97 = Subtract(x=w229, y=w228) -> (x-y=w232:i32)
                n98 = Array Subset(array=w230, index=w228, length=w232) -> (w231:dbl[])
                n99 = Array Max & Min(array=w231) -> (min value=w227:dbl)  [unwired: 3 out]
                n100 = property on="localMinima" class="DigNum (strict)"("Value"=w227) -> ()  [unwired: 2 in, 2 out]
              }
              frame #1 {
                n101 = property on="localMinima" class="DigNum (strict)"() -> ("Value"=w233:dbl)  [unwired: 2 in, 2 out]
                n102 = Number To Decimal String(number=w233) -> (decimal integer string=w235:string)  [unwired: 1 out]
                n103 = Concatenate Strings("DAC 2 " ("write buffer"), w235, "\n") -> (w234:string)
                n104 = VISA Write(VISA resource name=w239, write buffer=w234, error in (no error)=w238) -> ()  [unwired: 3 out]
              }
              frame #2 {
                n105 = call "Read MC Analog In.vi"("channel"=3) -> ("Voltage Input"=w241:dbl)  [unwired: 9 in, 1 out]
                n106 = Absolute Value(x=w241) -> (abs(x)=w244:dbl)
                n107 = property on="EndThresh" class="DigNum (strict)"() -> ("Value"=w242:dbl)  [unwired: 2 in, 2 out]
                n108 = Greater?(x=w244, y=w242) -> (0:w243:bool)
              }
            }
            n109 = Select(t="EXIT", s=w222, f="STAGE1-SWEEP") -> (s? t:f=w224:string)
          }
        }
        n110 = call "Convert to Dynamic Data"("Array"=w36) -> ("Dynamic Data Type"=w37:dynamicdata)  [unwired: 3 out]
        n111 = call "Convert to Dynamic Data2"("Array"=w35) -> ("Dynamic Data Type"=w38:dynamicdata)  [unwired: 3 out]
        n112 = call "Build XY Graph"("Y Input"=w38, "X Input"=w37) -> ("XY Graph"=→"XY Graph":cluster{"Y":dbl[], "Y":dbl[]}[])  [unwired: 3 in, 6 out]
      }
    }
    frame #3 {
      n113 = property on="Phase Voltage [v]" class="DigNum (strict)"() -> ("Value"=w247:dbl)  [unwired: 2 in, 2 out]
      n114 = VISA Close(VISA resource name=w249, error in (no error)=w248) -> ()  [unwired: 1 out]
      n115 = Bundle By Name(cluster=w246, "Phase Output Voltage [V]"=w247) -> (→"Hardware Parameters Out":T1)
    }
  }
